vi "SPARK Get Soft Limit Config.vi"   [LabVIEW 2023]
doc: "Get the configuration of a soft limit on the SPARK."
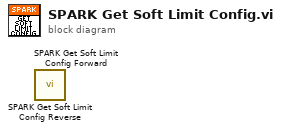
[diagram p0: block diagram]
diagram:
  n1 = call "SPARK Get Soft Limit Config Reverse.vi"() -> ()  [unwired: 8 in, 4 out]
  n2 = call "SPARK Get Soft Limit Config Forward.vi"() -> ()  [unwired: 8 in, 4 out]
